vi "Create.vi"(9 "External Result Ref":string, 10 "Summary":string, 11 "Outcome":T1) -> (3 "Test Run Result":refnum<class "Test Run Result.lvclass">)   [LabVIEW 2026, in "Test Run Result.lvclass"]
uses:
  Test Run Result.lvclass
  Test Run Result.lvclass/Test Run Result.ctl
  Typedefs/enums/Run Outcome Enum.ctl
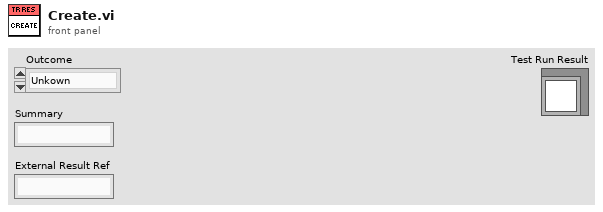
[diagram p1: front panel]
types:
  T1 = typedef "Run Outcome Enum.ctl" = enum16{"Unkown", "Passed", "Failed", "Error", "Aborted"}
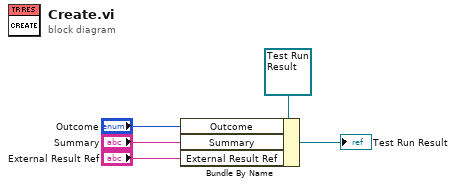
[diagram p0: block diagram]
diagram:
  n1 = Bundle By Name(cluster=refnum<class "Test Run Result.lvclass"> refnum ("Test Run Result.lvclass"), "Outcome"="Outcome", "Summary"="Summary", "External Result Ref"="External Result Ref") -> (→"Test Run Result":refnum<class "Test Run Result.lvclass">)
